vi "EFieldInStr.vi"(2 "Offset":dbl format="%.1f", 3 "read buffer":string, 4 "controllo_segno":bool) -> (0 "kV/m":string, 1 "mV":string)   [LabVIEW 2010]
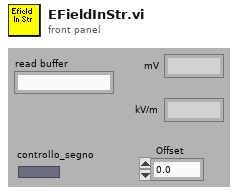
[diagram p1: front panel]
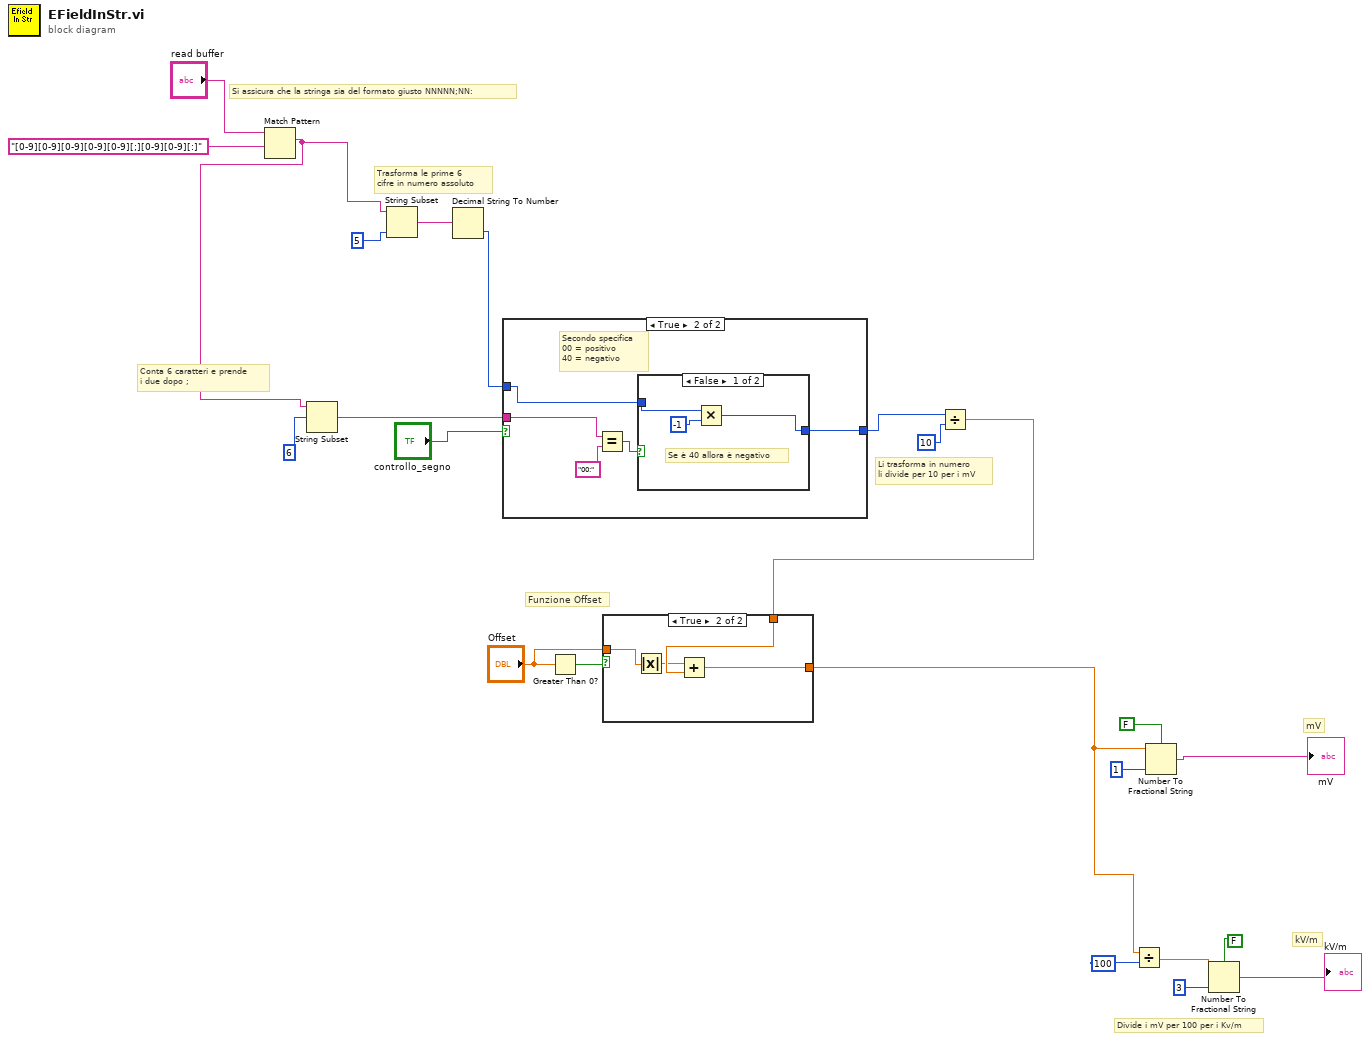
[diagram p0: block diagram]
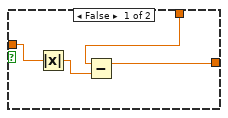
[diagram p2: hidden frame]
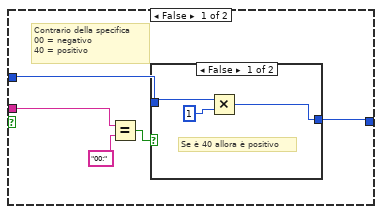
[diagram p3: hidden frame]
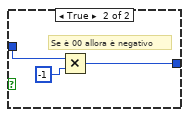
[diagram p4: hidden frame]
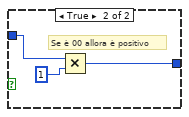
[diagram p5: hidden frame]
diagram:
  # "kV/m"
  # "mV"
  # "Funzione Offset"
  # "Li trasforma in numero\nli divide per 10 per i mV"
  # "Trasforma le prime 6\ncifre in numero assoluto"
  # "Divide i mV per 100 per i Kv/m"
  # "Conta 6 caratteri e prende\ni due dopo ;"
  # "Si assicura che la stringa sia del formato giusto NNNNN;NN:"
  n1 = Match Pattern(string="read buffer", regular expression="[0-9][0-9][0-9][0-9][0-9][;][0-9][0-9][:]" ("format string")) -> (match substring=w10:string)  [unwired: 1 in, 3 out]
  n2 = String Subset(string=w10, offset (0)=6) -> (substring=w8:string)  [unwired: 1 in]
  n3 = String Subset(string=w10, length (rest)=5) -> (substring=w15:string)  [unwired: 1 in]
  n4 = Decimal String To Number(string=w15) -> (number=w7:i32)  [unwired: 2 in, 1 out]
  n5 = case shown="True" "controllo_segno" {
    tunnel: w8 -> [w26 w38]
    tunnel: w7 -> [w25 w35]
    tunnel: [w24 w36] -> w6
    frame False {
      # "Contrario della specifica\n00 = negativo\n40 = positivo"
      n6 = Equal?(x=w26, y="00:") -> (x = y?=w27:bool)
      n7 = case shown="False" w27 {
        tunnel: w25 -> [w30 w33]
        tunnel: [w29 w32] -> w24
        frame False {
          # "Se è 40 allora è positivo"
          n8 = Multiply(x=w30, y=1) -> (x*y=w29:i32)
        }
        frame True {
          # "Se è 00 allora è negativo"
          n9 = Multiply(x=w33, y=-1) -> (x*y=w32:i32)
        }
      }
    }
    frame True {
      # "Secondo specifica\n00 = positivo\n40 = negativo"
      n10 = Equal?(x=w38, y="00:") -> (x = y?=w37:bool)
      n11 = case shown="False" w37 {
        tunnel: w35 -> [w41 w43]
        tunnel: [w40 w44] -> w36
        frame False {
          # "Se è 40 allora è negativo"
          n12 = Multiply(x=w41, y=-1) -> (x*y=w40:i32)
        }
        frame True {
          # "Se è 00 allora è positivo"
          n13 = Multiply(x=w43, y=1) -> (x*y=w44:i32)
        }
      }
    }
  }
  n14 = Greater Than 0?(x="Offset") -> (x > 0?=w4:bool)
  n15 = Divide(x=w6, y=10) -> (x/y=w2:dbl)
  n16 = case shown="True" w4 {
    tunnel: "Offset" -> [w46 w53]
    tunnel: w2 -> [w49 w52]
    tunnel: [w47 w50] -> w1
    frame False {
      n17 = Absolute Value(x=w46) -> (abs(x)=w48:dbl)
      n18 = Subtract(x=w49, y=w48) -> (x-y=w47:dbl)
    }
    frame True {
      n19 = Absolute Value(x=w53) -> (abs(x)=w51:dbl)
      n20 = Add(x=w51, y=w52) -> (x+y=w50:dbl)
    }
  }
  n21 = Divide(x=w1, y=100) -> (x/y=w21:dbl)
  n22 = Number To Fractional String(use system decimal point (T)=FALSE, number=w1, precision (6)=1) -> (F-format string=→"mV":string)  [unwired: 1 in]
  n23 = Number To Fractional String(use system decimal point (T)=FALSE, number=w21, precision (6)=3) -> (F-format string=→"kV/m":string)  [unwired: 1 in]
